vi "CPP-6342ApproxEfficiency.vi"() -> (5 "Plug in titles":string[](array[string]), 7 "Plug in values":string[](array[string]))   [LabVIEW 2012]
uses:
  Globals/Meas_global.vi
  CPP/ProjectSpecific/6342-IESWindTurbine/RPMGlobal.vi
panel:
  out "TipSpeedRatio":dbl format="%.2f"
  out "Cp(%)":dbl format="%.1f"
  out "RotorPower(Watts)":dbl format="%.1f"
  out "StreamPower(Watts)":dbl format="%.1f"
  out "Torque(N-m)":dbl format="%.2f"
  out "WindSpeed(m/s)":dbl format="%.1f"
  in  "RotorDiameter(in)":dbl=40.0
  # "!!Pitot on 0, Torque on 1, & RPM vi must be running!!"
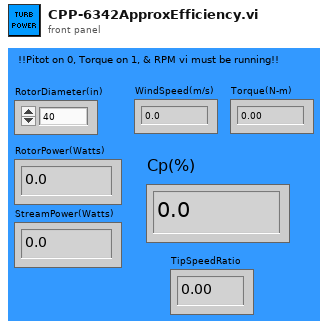
[diagram p1: front panel]
types:
  T1 = typedef "Analysis_info_cluster.ctl" = cluster{"Colour":u32, "Inst type":T2, "Inst name":string, "Symbol":string, "Code name":string, "Extra Info":string, "Inst Array":T3, "Extra Titles":string[], "Extra Values":string[], "U":dbl, "u^2":dbl, "u^3":dbl, "u^4":dbl, "Skew_u":dbl, "Kurt_u":dbl, "Sd Error in Mean":dbl, "% u'/U":dbl, "X":dbl, "Y":dbl, "Z":dbl, "Timescale integral to 25%":dbl, "Sd Error in Variance":dbl, "Calib File":path, "Calib Constants":dbl[], "Output Position":bool, "Full Stats":bool, "Av Sampling Rate":dbl, "Av No of Samples":dbl, "Total Meas Time (s)":dbl, "ADAM Ch Name":string}
  T2 = typedef "Inst_type.ctl" = enum16{"Propeller anemometer", "Raw voltage", "Pressure Transducer", "Pitot-static tube", "Preston tube", "Hot wire", "Cross wire 1", "Cross wire 2", "Generic Linear", "Generic Polynomial", "Generic BackPoly", "Fast FID", "Thermocouple", "Cold wire", "Pulsed Wire", "LDA Vel", "LDA Tran time", "LDA Arr time"}
  T3 = typedef "Instrument_Array.ctl" = enum16{"PWA", "LDA", "Analogue"}
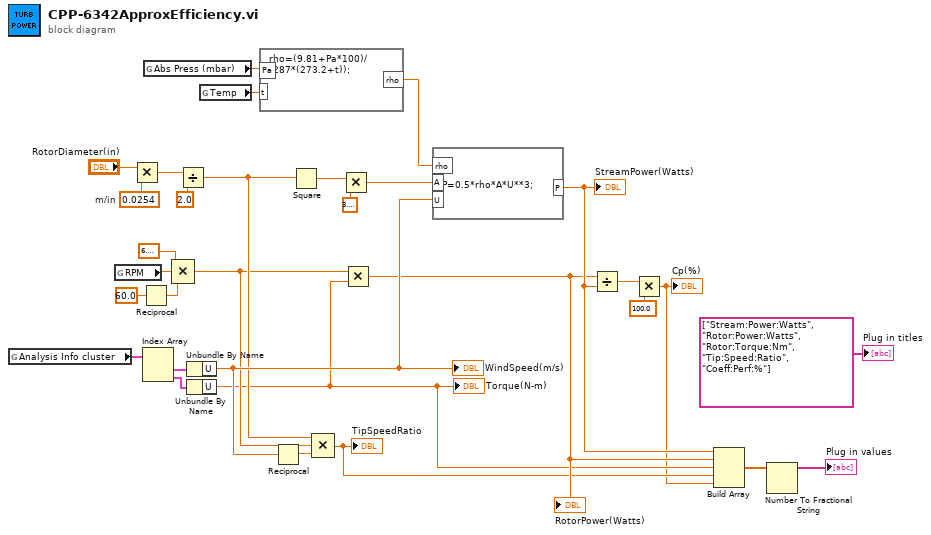
[diagram p0: block diagram]
diagram:
  w22 = 0.0254  # m/in
  n1 = global read "Meas_global.vi" "Analysis Info cluster"() -> (w31:T1[])
  n2 = global read "RPMGlobal.vi" "RPM"() -> (w17:dbl)
  n3 = Multiply(x="RotorDiameter(in)", y=w22) -> (x*y=w18:dbl)
  n4 = Reciprocal(x=60.0 ("y")) -> (1/x=w16:dbl)
  n5 = Index Array(array=w31) -> (element #1=w30:T1, element #2=w29:T1)  [unwired: 2 in]
  n6 = global read "Meas_global.vi" "Abs Press (mbar)"() -> (w28:dbl)
  n7 = Compound Arithmetic op=MULTIPLY(6.283185307179586, w17, w16) -> (w13:dbl)
  n8 = Divide(x=w18, y=2.0) -> (x/y=w14:dbl)
  n9 = Unbundle By Name(w30) -> ("U"=w15:dbl)
  "WindSpeed(m/s)" <- w15
  n10 = Unbundle By Name(w29) -> ("U"=w5:dbl)
  "Torque(N-m)" <- w5
  n11 = global read "Meas_global.vi" "Temp"() -> (w27:dbl)
  n12 = formula code="rho=(9.81+Pa*100)/\n(287*(273.2+t));"("t"=w27, "Pa"=w28) -> ("rho"=w26:dbl)
  n13 = Reciprocal(x=w15) -> (1/x=w12:dbl)
  n14 = Square(x=w14) -> (x^2=w25:dbl)
  n15 = Compound Arithmetic op=MULTIPLY(w14, w13, w12) -> (w4:dbl)
  "TipSpeedRatio" <- w4
  n16 = Multiply(x=w25, y=3.141592653589793) -> (x*y=w24:dbl)
  n17 = Multiply(x=w13, y=w5) -> (x*y=w6:dbl)
  "RotorPower(Watts)" <- w6
  n18 = formula code="P=0.5*rho*A*U**3;"("A"=w24, "rho"=w26, "U"=w15) -> ("P"=w7:dbl)
  "StreamPower(Watts)" <- w7
  n19 = Divide(x=w6, y=w7) -> (x/y=w20:dbl)
  n20 = Multiply(x=w20, y=100.0) -> (x*y=w3:dbl)
  "Cp(%)" <- w3
  n21 = Build Array(w7, w6, w5, w4, w3) -> (w2:dbl[])
  n22 = Number To Fractional String(number=w2) -> (F-format string=→"Plug in values":string[])  [unwired: 3 in]
  "Plug in titles" <- string[] ["Stream:Power:Watts", "Rotor:Power:Watts", "Rotor:Torque:Nm", "Tip:Speed:Ratio", "Coeff:Perf:%"] ("Plug in titles")
